vi "Prepare Get Recipe JSON.vi"(10 "Run.Start JSON":string="{\n  \"id\": \"9f3c1ab2e4d5\",\n  \"op\": \"run.start\",\n  \"args\": {\n    \"run_id\": \"7b1e0c9a8f24\",\n    \"recipe_id\": \"INV\",\n    \"version\": 1,\n    \"run_parameters\": {\n      \"barcode\": \"INV12345\",\n      \"serial_no\": \"INV12345\",\n      \"model\": \"INV\"\n    }\n  },\n  \"reply_to\": \"tmf/st1/cmd/resp/tmf-py-1a2b3c4d\"\n}") -> (2 "resulting string":string)   [LabVIEW 2021, in "Sequence Engine.lvlib"]
uses:
  d02a36d8-32d7-4c34-840c-d876fb744b65.vi
  2bc376ff-0326-4313-8969-65efc966226b.vi
  904c2c43-94fe-4a76-a9d7-c6b690628e6e.vi
  df84fae3-b476-4c4c-9a4e-dd2ee642f6f0.vi
  4e0d7212-e0d4-47ba-b0b7-f44cdc49669f.vi
  <vilib>/JDP Science/JSONtext/Find Item.vi
  <vilib>/JDP Science/JSONtext/Next JSON Value.vi
  <vilib>/JDP Science/JSONtext/String Subset.vi
  <vilib>/JDP Science/JSONtext/Parsing/Advance past next JSON Value (inlined COPY).vi
  <vilib>/JDP Science/JSONtext/Parsing/Advance past whitespace.vi
  <vilib>/JDP Science/JSONtext/Parsing/Advance past String.vi
  <vilib>/JDP Science/JSONtext/Parsing/Advance past Number.vi
  <vilib>/JDP Science/JSONtext/Parsing/Advance past Line Ending.vi
  <vilib>/JDP Science/JSONtext/Parsing/Parse Full Path or Item Name.vi
  <vilib>/JDP Science/JSONtext/Parsing/Advance past Array.vi
  <vilib>/JDP Science/JSONtext/Parsing/Advance past Object.vi
  <vilib>/JDP Science/JSONtext/support/Error Cluster From Code.vi
  <vilib>/JDP Science/JSONtext/Offset/Find Item Locations by Path.vi
  <vilib>/JDP Science/JSONtext/JSON text to Variant.vi
  <vilib>/JDP Science/JSONtext/LVClass Serializer/JSONtext LVClass Serializer.lvclass
  Sequence Engine.lvlib
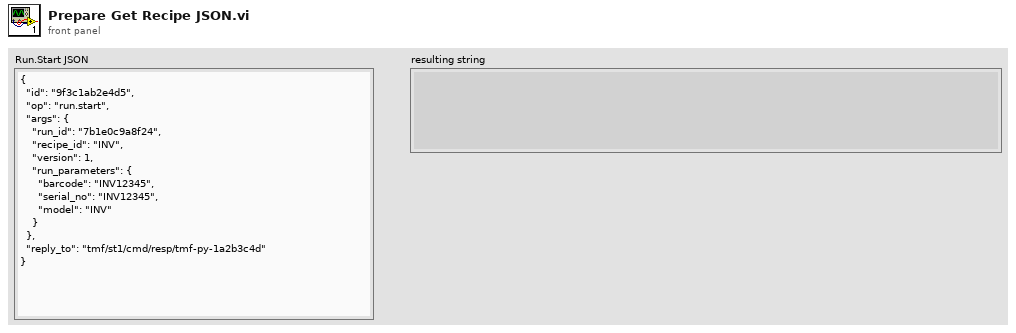
[diagram p1: front panel]
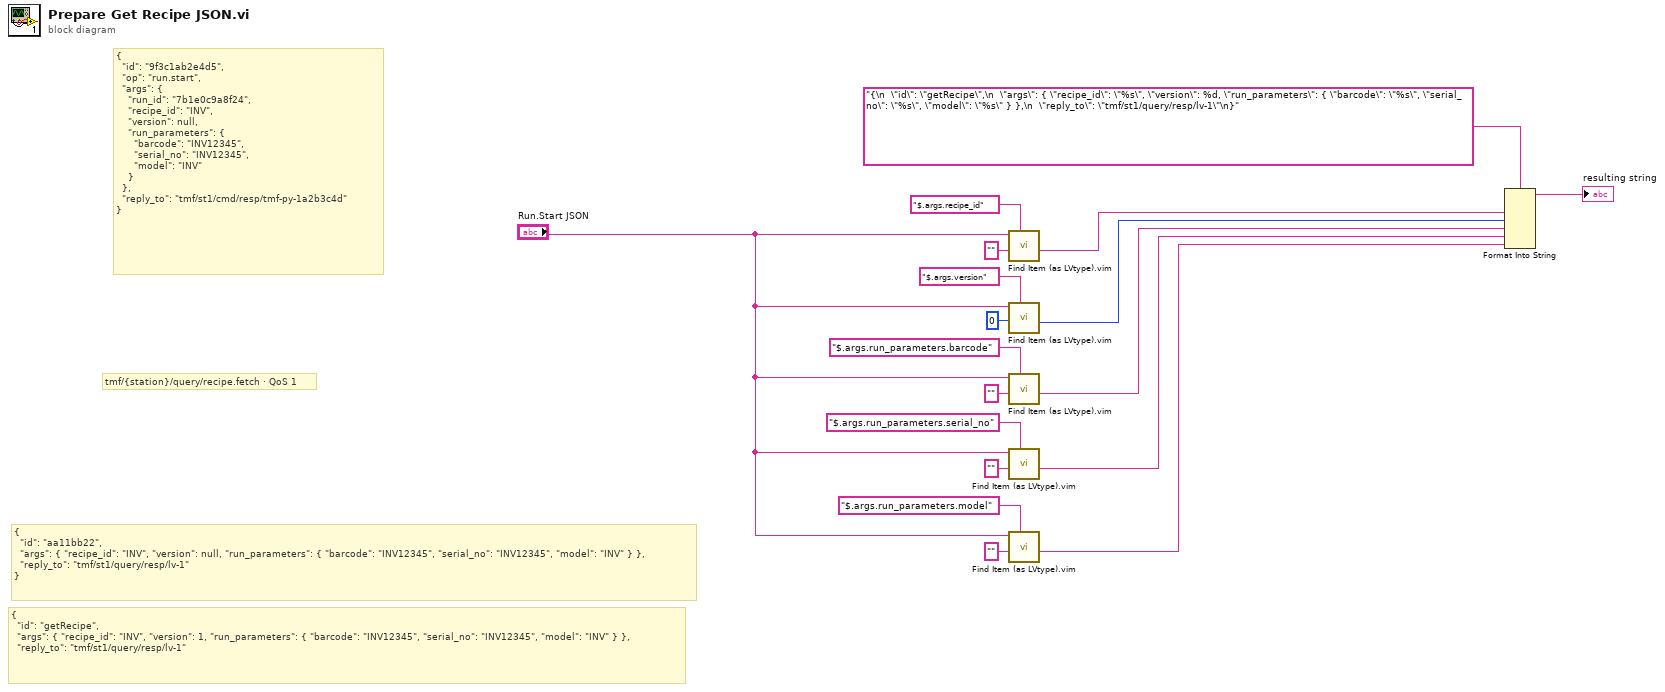
[diagram p0: block diagram]
diagram:
  # "{\n  \"id\": \"getRecipe\",\n  \"args\": { \"recipe_id\": \"INV\", \"version\": 1, \"run_parameters\": { \"barcode\": \"INV12345\", \"serial_no\": \"INV12345\", \"model\": \"INV\" } },\n  \"reply_to\": \"tmf/st1/query/resp/lv-1\""
  # "tmf/{station}/query/recipe.fetch · QoS 1"
  # "{\n  \"id\": \"aa11bb22\",\n  \"args\": { \"recipe_id\": \"INV\", \"version\": null, \"run_parameters\": { \"barcode\": \"INV12345\", \"serial_no\": \"INV12345\", \"model\": \"INV\" } },\n  \"reply_to\": \"tmf/st1/query/resp/lv-1\"\n}"
  # "{\n  \"id\": \"9f3c1ab2e4d5\",\n  \"op\": \"run.start\",\n  \"args\": {\n    \"run_id\": \"7b1e0c9a8f24\",\n    \"recipe_id\": \"INV\",\n    \"version\": null,\n    \"run_parameters\": {\n      \"barcode\": \"INV12345\",\n      \"serial_no\": \"INV12345\",\n      \"model\": \"INV\"\n    }\n  },\n  \"reply_to\": \"tmf/st1/cmd/resp/tmf-py-1a2b3c4d\"\n}"
  n1 = call "Find Item (as LVtype).vim"("$Path or Item Name"="$.args.recipe_id", "Data Type and Default Value"="", "JSON"="Run.Start JSON") -> ("Data"=w15:string)  [unwired: 5 in, 3 out]
  n2 = call "Find Item (as LVtype).vim"("$Path or Item Name"="$.args.version", "Data Type and Default Value"=0, "JSON"="Run.Start JSON") -> ("Data"=w12:i32)  [unwired: 5 in, 3 out]
  n3 = call "Find Item (as LVtype).vim"("$Path or Item Name"="$.args.run_parameters.barcode", "Data Type and Default Value"="", "JSON"="Run.Start JSON") -> ("Data"=w9:string)  [unwired: 5 in, 3 out]
  n4 = call "Find Item (as LVtype).vim"("$Path or Item Name"="$.args.run_parameters.serial_no", "Data Type and Default Value"="", "JSON"="Run.Start JSON") -> ("Data"=w6:string)  [unwired: 5 in, 3 out]
  n5 = call "Find Item (as LVtype).vim"("$Path or Item Name"="$.args.run_parameters.model", "Data Type and Default Value"="", "JSON"="Run.Start JSON") -> ("Data"=w2:string)  [unwired: 5 in, 3 out]
  n6 = Format Into String(format string="{\n  \"id\": \"getRecipe\",\n  \"args\": { \"recipe_id\": \"%s\", \"version\": %d, \"run_parameters\": { \"barcode\": \"%s\", \"serial_no\": \"%s\", \"model\": \"%s\" } },\n  \"reply_to\": \"tmf/st1/query/resp/lv-1\"\n}", w15, w12, w9, w6, w2) -> (resulting string=→"resulting string":string)  [unwired: 2 in, 1 out]
